vi "Bool.vi"() -> ()   [LabVIEW 2018]
panel:
  in  "Boolean":bool
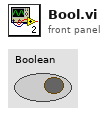
[diagram p1: front panel]
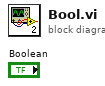
[diagram p0: block diagram]
diagram:
